vi "Write Update Msg.vi"(6 "Update Active Attribute Value Msg":refnum<class "Update Active Attribute Value Msg.lvclass">, 11 "IAttribute Data Type View in":refnum<class "IAttribute Data Type View.lvclass">) -> (3 "IAttribute Data Type View out":refnum<class "IAttribute Data Type View.lvclass">)   [LabVIEW 2017]
uses:
  IAttribute Data Type View.lvclass
  C:/Users/jonmc/Documents/Git/Test Executive Builder/gpm_packages/@cs/mva-framework/Source/Framework/IViewable/IViewable/IViewable.lvclass
  C:/Users/jonmc/Documents/Git/Test Executive Builder/gpm_packages/@cs/mva-framework/Source/Framework/ActorEvents/IEventAggregator/IEventAggregator.lvclass
  C:/Users/jonmc/Documents/Git/Test Executive Builder/gpm_packages/@cs/mva-framework/Source/Framework/IObserver/IObserver/IObserver.lvclass
  C:/Program Files (x86)/National Instruments/LabVIEW 2017/vi.lib/ActorFramework/Actor/Actor.lvclass
  ITest Executive Builder Dialog Messages/Update Active Attribute Value Msg/Update Active Attribute Value Msg.lvclass
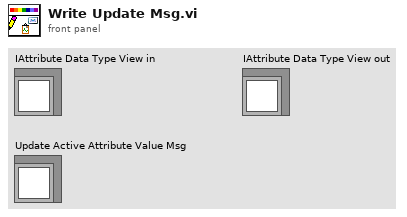
[diagram p1: front panel]
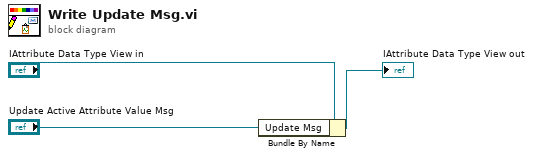
[diagram p0: block diagram]
diagram:
  n1 = Bundle By Name(cluster="IAttribute Data Type View in", "Update Msg"="Update Active Attribute Value Msg") -> (→"IAttribute Data Type View out":refnum<class "IAttribute Data Type View.lvclass">)
